vi "TharOn.vi"(8 "Error In":errorcluster, 11 "Device Serial Number":string) -> (0 "Error Out":errorcluster, 3 "Device Serial Number Out":string)   [LabVIEW 2016]
panel:
  out "Bytes Written":u32
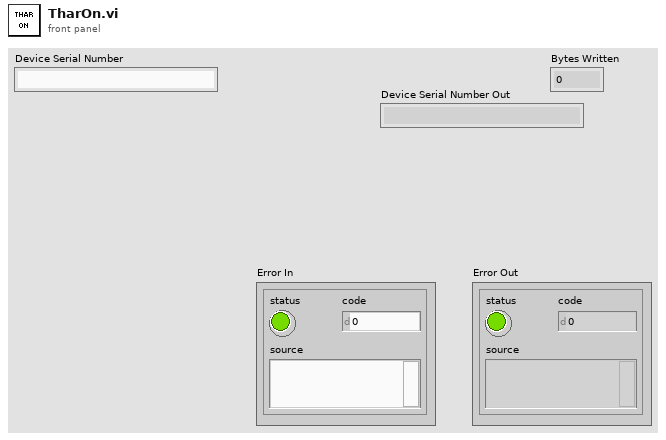
[diagram p1: front panel]
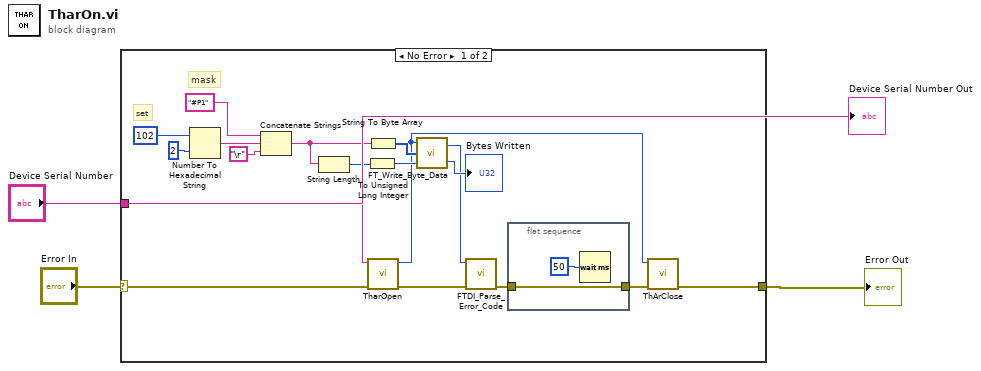
[diagram p0: block diagram]
diagram:
  n1 = case shown="No Error" "Error In" {
    selector: "Error In" -> [w4 w24]
    tunnel: "Device Serial Number" -> [w13 _]
    tunnel: [w10 w24] -> w2
    frame No Error {
      # "set"
      # "mask"
      n2 = Number To Hexadecimal String(1:i16 2 ("width (-)"), 2:102 ("number")) -> (0:w20:string)
      n3 = Concatenate Strings("#P1" ("Substring"), w20, "\r") -> (w14:string)
      n4 = String Length(string=w14) -> (length=w18:i32)
      n5 = To Unsigned Long Integer(number=w18) -> (unsigned 32bit integer=w17:u32)
      n6 = String To Byte Array(string=w14) -> (unsigned byte array=w16:u8[])
      n7 = call "TharOpen.vi"("error in (no error)"=w4, "Device Serial Number"=w13) -> ("error constant"=w9:errorcluster, "Handle"=w11:u32)  [unwired: 8 in]
      n8 = call "FT_Write_Byte_Data.vi"("Bytes To Write"=w17, "Buffer"=w16, "Handle"=w11) -> ("Bytes Written"=→"Bytes Written":u32, "FT_Status"=w12:u32)
      n9 = call "FTDI_Parse_Error_Code.vi"("error in (no error)"=w9, "FT_Status"=w12) -> ("error out"=w8:errorcluster)  [unwired: 9 in]
      n10 = flat-sequence {
        tunnel: w8 -> [w22]
        tunnel: [w22] -> w7
        frame #0 {
          n11 = Wait (ms)(milliseconds to wait=u32 50) -> ()  [unwired: 1 out]
        }
      }
      n12 = call "ThArClose.vi"("error in (no error)"=w7, "Handle"=w11) -> ("error out"=w10:errorcluster)  [unwired: 9 in]
    }
    frame Error {
    }
  }
  "Error Out" <- w2
  "Device Serial Number Out" <- "Device Serial Number"
